vi "SineWaveLoop.vi"() -> ()   [LabVIEW 2019]
panel:
  out "A*sin(2pift+theta)":dbl[](graph)=[0.0, 0.06279051952931337, 0.12533323356430426, 0.1873813145857246, 0.2486898871648548, 0.3090169943749474, 0.3681245526846779, 0.42577929156507266, 0.4817536741017153, 0.5358267949789967, 0.5877852522924731, 0.6374239897486897, 0.6845471059286886, 0.7289686274214116, 0.7705132427757893, 0.8090169943749475, 0.8443279255020151, 0.8763066800438636, 0.9048270524660196, 0.9297764858882515, 0.9510565162951535, 0.9685831611286311, 0.9822872507286887, 0.9921147013144779, 0.9980267284282716, 1.0, 0.9980267284282716, 0.9921147013144778, 0.9822872507286887, 0.9685831611286312, 0.9510565162951535, 0.9297764858882515, 0.9048270524660195, 0.8763066800438635, 0.8443279255020152, 0.8090169943749475, 0.7705132427757893, 0.7289686274214114, 0.6845471059286885, 0.6374239897486899, 0.5877852522924732, 0.5358267949789962, 0.4817536741017152, 0.4257792915650725, 0.36812455268467775, 0.3090169943749475, 0.24868988716485482, 0.18738131458572457, 0.12533323356430454, 0.06279051952931358, 1.2246467991473532e-16, -0.06279051952931378, -0.12533323356430429, -0.18738131458572477, -0.24868988716485502, -0.3090169943749473, -0.3681245526846779, -0.42577929156507266, -0.481753674101715, -0.5358267949789964, -0.5877852522924734, -0.63742398974869, -0.6845471059286887, -0.7289686274214116, -0.7705132427757894, -0.8090169943749473, -0.8443279255020153, -0.8763066800438636, -0.9048270524660194, -0.9297764858882515, -0.9510565162951535, -0.9685831611286312, -0.9822872507286887, -0.9921147013144778, -0.9980267284282716, -1.0, -0.9980267284282716, -0.9921147013144779, -0.9822872507286887, -0.9685831611286311, -0.9510565162951536, -0.9297764858882516, -0.9048270524660191, -0.8763066800438634, -0.844327925502015, -0.809016994374947, -0.770513242775789, -0.7289686274214116, -0.6845471059286883, -0.6374239897486896, -0.5877852522924734, -0.5358267949789963, -0.4817536741017153, -0.425779291565073, -0.36812455268467786, -0.3090169943749477, -0.24868988716485535, -0.18738131458572468, -0.12533323356430465, -0.06279051952931326, -2.4492935982947064e-16, 0.06279051952931278, 0.12533323356430506, 0.18738131458572507, 0.24868988716485488, 0.309016994374948, 0.3681245526846782, 0.42577929156507255, 0.48175367410171566, 0.5358267949789967, 0.5877852522924729, 0.63742398974869, 0.6845471059286886, 0.7289686274214112, 0.7705132427757893, 0.8090169943749472, 0.8443279255020147, 0.8763066800438636, 0.9048270524660194, 0.9297764858882518, 0.9510565162951538, 0.9685831611286312, 0.9822872507286888, 0.9921147013144779, 0.9980267284282716, 1.0, 0.9980267284282716, 0.9921147013144779, 0.9822872507286886, 0.9685831611286311, 0.9510565162951536, 0.929776485888251, 0.9048270524660192, 0.8763066800438634, 0.8443279255020151, 0.8090169943749476, 0.7705132427757897, 0.728968627421411, 0.6845471059286884, 0.6374239897486897, 0.5877852522924734, 0.5358267949789972, 0.48175367410171466, 0.4257792915650723, 0.368124552684678, 0.3090169943749478, 0.2486898871648555, 0.18738131458572568, 0.1253332335643039, 0.06279051952931339, 3.6739403974420594e-16, -0.06279051952931443, -0.12533323356430492, -0.18738131458572496, -0.24868988716485477, -0.30901699437494706, -0.36812455268467725, -0.42577929156507166, -0.48175367410171555, -0.5358267949789965, -0.5877852522924728, -0.6374239897486892, -0.6845471059286878, -0.7289686274214106, -0.7705132427757904, -0.8090169943749482, -0.8443279255020156, -0.8763066800438639, -0.9048270524660197, -0.9297764858882507, -0.951056516295154, -0.9685831611286314, -0.9822872507286888, -0.9921147013144779, -0.9980267284282716, -1.0, -0.9980267284282714, -0.9921147013144778, -0.9822872507286886, -0.9685831611286312, -0.9510565162951538, -0.929776485888251, -0.9048270524660192, -0.8763066800438635, -0.8443279255020152, -0.8090169943749477, -0.7705132427757898, -0.7289686274214111, -0.6845471059286885, -0.6374239897486897, -0.5877852522924735, -0.5358267949789973, -0.4817536741017163, -0.42577929156507244, -0.3681245526846781, -0.3090169943749479, -0.2486898871648556, -0.1873813145857258, -0.125333233564304, -0.06279051952931351, -4.898587196589413e-16, 0.06279051952931253, 0.12533323356430304, 0.1873813145857231, 0.24868988716485638, 0.3090169943749486, 0.3681245526846788, 0.42577929156507316, 0.48175367410171543, 0.5358267949789964, 0.5877852522924741, 0.6374239897486904, 0.6845471059286891, 0.7289686274214117, 0.7705132427757891, 0.8090169943749471, 0.8443279255020155, 0.8763066800438638, 0.9048270524660196, 0.9297764858882513, 0.9510565162951534, 0.9685831611286313, 0.9822872507286888, 0.9921147013144779, 0.9980267284282716, 1.0, 0.9980267284282717, 0.9921147013144778, 0.9822872507286886, 0.9685831611286312, 0.9510565162951538, 0.9297764858882518, 0.9048270524660201, 0.8763066800438635, 0.8443279255020152, 0.8090169943749478, 0.7705132427757898, 0.7289686274214124, 0.6845471059286873, 0.6374239897486885, 0.5877852522924721, 0.5358267949789959, 0.4817536741017149, 0.42577929156507255, 0.36812455268467653, 0.3090169943749463, 0.248689887164854, 0.18738131458572418, 0.12533323356430415, 0.06279051952931362, -1.164033439826574e-15, -0.06279051952931418, -0.1253332335643047, -0.1873813145857247, -0.24868988716485452, -0.3090169943749451, -0.3681245526846787, -0.42577929156507305, -0.4817536741017153, -0.5358267949789963, -0.5877852522924726, -0.6374239897486917, -0.6845471059286903, -0.7289686274214128, -0.7705132427757901, -0.8090169943749481, -0.8443279255020155, -0.8763066800438638, -0.9048270524660196, -0.9297764858882513, -0.9510565162951534, -0.9685831611286309, -0.9822872507286884, -0.9921147013144781, -0.9980267284282717, -1.0, -0.9980267284282716, -0.9921147013144778, -0.9822872507286887, -0.9685831611286312, -0.9510565162951538, -0.9297764858882518, -0.9048270524660201, -0.8763066800438645, -0.8443279255020143, -0.8090169943749468, -0.7705132427757888, -0.7289686274214113, -0.6845471059286886, -0.63742398974869, -0.5877852522924737, -0.5358267949789975, -0.48175367410171654, -0.42577929156507427, -0.36812455268468, -0.3090169943749498, -0.2486898871648541, -0.1873813145857243, -0.12533323356430426, -0.06279051952931375]
  out "No. of\nsamples":dbl=300.0
  in  "No. of\ncycles":dbl=3.0
  in  "fs":dbl=10000.0
  in  "Phase":dbl
  in  "f":dbl=100.0
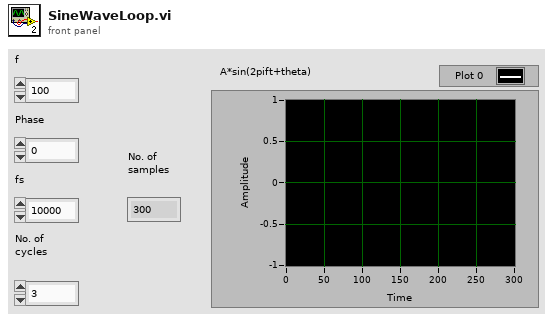
[diagram p1: front panel]
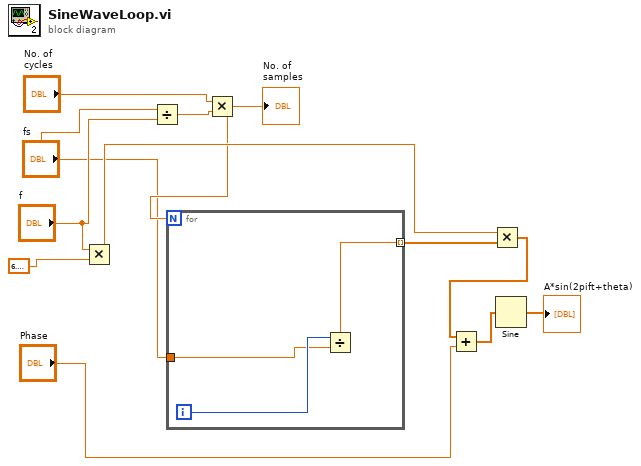
[diagram p0: block diagram]
diagram:
  n1 = Multiply(x="f", y=6.283185307179586) -> (x*y=w12:dbl)
  n2 = Divide(x="fs", y="f") -> (x/y=w7:dbl)
  n3 = Multiply(x="No. of\ncycles", y=w7) -> (x*y=w5:dbl)
  "No. of\nsamples" <- w5
  n4 = for {
    N: w5 -> [_]
    tunnel: [w15] -> w4 mode=indexing
    tunnel: "fs" -> [w13]
    i -> [w14]
    n5 = Divide(x=w14, y=w13) -> (x/y=w15:dbl)
  }
  n6 = Multiply(x=w12, y=w4) -> (x*y=w9:dbl[])
  n7 = Add(x=w9, y="Phase") -> (x+y=w10:dbl[])
  n8 = Sine(x=w10) -> (sin(x)=→"A*sin(2pift+theta)":dbl[])
